vi "Delete Items (inline).vi"(6 "indent":i32, 8 "error in (no error)":errorcluster, 9 "Copy? (F)":bool, 10 "Indices to remove":i32[](array[numeric]), 11 "BetterHandle in":refnum<class "BetterHandle.lvclass">) -> (0 "error out":errorcluster, 2 "items removed":refnum<class "BetterItem.lvclass">[](array[class]), 3 "BetterHandle out":refnum<class "BetterHandle.lvclass">)   [LabVIEW 2020, in "BetterDragAndDrop.lvlib" / "BetterHandle.lvclass"]
uses:
  BetterHandle.lvclass
  BetterTreeItem/BetterItem.lvclass
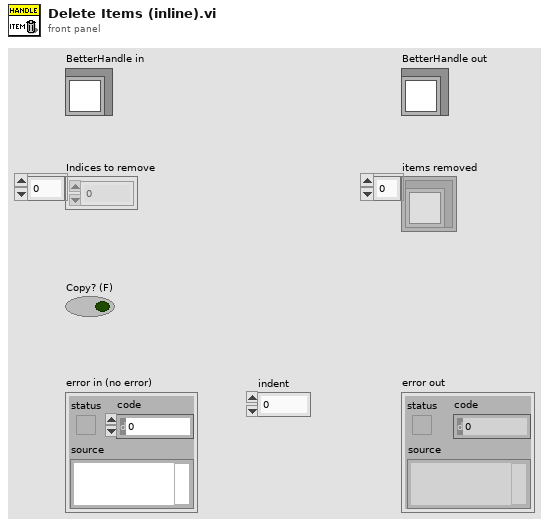
[diagram p1: front panel]
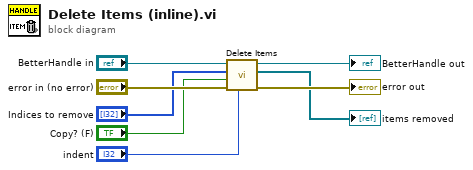
[diagram p0: block diagram]
diagram:
  n1 = call-dynamic "Delete Items.vi"("indent"="indent", "error in (no error)"="error in (no error)", "Copy? (F)"="Copy? (F)", "Indices to remove"="Indices to remove", "BetterHandle in"="BetterHandle in") -> ("error out"=→"error out":errorcluster, "items removed"=→"items removed":refnum<class "BetterItem.lvclass">[], "BetterHandle out"=→"BetterHandle out":refnum<class "BetterHandle.lvclass">)  [unwired: 4 in]
